vi "Protocol status-idle.vi"   [LabVIEW 2020]
uses:
  General Globals.vi
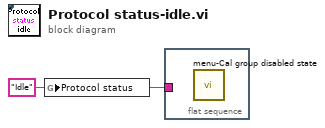
[diagram p0: block diagram]
diagram:
  w1 = "Idle" ("Protocol status")
  n1 = global write "General Globals.vi" "Protocol status"(w1) -> ()
  n2 = flat-sequence {
    tunnel: w1 -> [_]
    frame #0 {
      n3 = call "menu-Cal group disabled state.vi"() -> ()  [unwired: 10 in, 2 out]
    }
  }
